vi "ArcadeDriveTest.vi"() -> ()   [LabVIEW 2013]
uses:
  <vilib>/Rock Robotics/WPI/Joystick/WPI_JoystickDeviceEnum.ctl
  <vilib>/Rock Robotics/SystemInterfaces/DIO/FPGA_DIOPWMChannel.ctl
  <vilib>/Rock Robotics/WPI/RobotDrive/WPI_RobotDriveOpen4MotorWithTalon.vi
  ArcadeDrivePieceWise.vi
  <vilib>/Rock Robotics/WPI/RobotDrive/WPI_RobotDriveArcadeDrive_RatioCurve.vi
panel:
  in  "Cutoff":dbl=0.7 format="%#_13g"
  in  "Deadzone":dbl=0.05 format="%#_13g"
  in  "UseWPILib?":bool
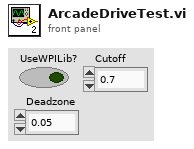
[diagram p1: front panel]
types:
  T1 = typedef "FPGA_DIOPWMChannel.ctl" = enum8{"PWM 1", "PWM 2", "PWM 3", "PWM 4", "PWM 5", "PWM 6", "PWM 7", "PWM 8", "PWM 9", "PWM 10", "Invalid"}
  T2 = typedef "WPI_JoystickDeviceEnum.ctl" = enum16{"USB 1", "USB 2", "USB 3", "USB 4", "Kinect 1", "Kinect 2"}
  T3 = typedef "WPI_RobotDriveDevRef.ctl" = cluster{"DevStatus":errorcluster, "Motors[]":T4[], "Square Inputs":bool, "Max Output":dbl, "Isochronous":bool}
  T4 = typedef "WPI_MotorControlDeviceRef.ctl" = cluster{"DeviceStatus":errorcluster, "Type":enum16{"PWM", "CAN"}, "PWM":cluster{"Digital Module":T5, "PWM Channel":T1, "DeadBand":T6}, "CAN":cluster{"Device Number":u8, "Control Mode":T7, "Semaphore":T8, "Max Vout":dbl}, "Invert":bool, "TransformRef":T9, "InvTransformRef":T9}
  T5 = typedef "FPGA_TypedefDigitalModule.ctl" = enum16{"Digital Module 1", "Digital Module 2"}
  T6 = typedef "WPI_PWMDeadband.ctl" = cluster{"Name":string, "maxPositivePwm":i32, "minPositivePwm":i32, "centerPwm":i32, "maxNegativePwm":i32, "minNegativePwm":i32, "angularRange":u16}
  T7 = typedef "WPI_CANJaguar_ControlMode.ctl" = enum8{"Percent VBus", "Current", "Speed", "Position", "Voltage"}
  T8 = typedef "Semaphore RefNum" = refnum<k1>
  T9 = typedef "WPI_PWMTransform_ConPane.ctl" = refnum<vi>
  T10 = typedef "WPI_JoystickDevRef.ctl" = cluster{"Device":T2}
  T11 = cluster{"axis 1 (x)":dbl, "axis 2 (y)":dbl, "axis 3 (throttle)":dbl, "axis 4":dbl, "axis 5":dbl, "axis 6":dbl}
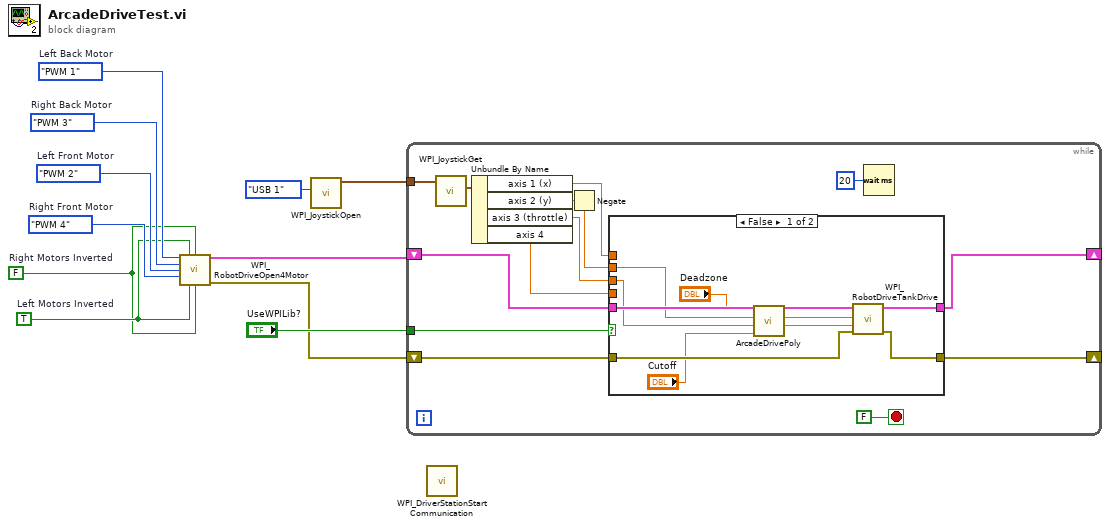
[diagram p0: block diagram]
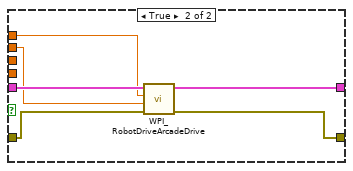
[diagram p2: hidden frame]
diagram:
  w5 = FPGA_DIOPWMChannel."PWM 4"  # Right Front Motor
  w6 = FPGA_DIOPWMChannel."PWM 2"  # Left Front Motor
  w7 = FPGA_DIOPWMChannel."PWM 3"  # Right Back Motor
  w8 = FPGA_DIOPWMChannel."PWM 1"  # Left Back Motor
  w3 = FALSE  # Right Motors Inverted
  w4 = TRUE  # Left Motors Inverted
  n1 = call-poly <vilib>:"WPI_RobotDriveOpen4Motor.vi"("Rear Left Motor"=w8, "Rear Left Motor Inverted"=w4, "Rear Right Motor Inverted"=w3, "Rear Right Motor"=w7, "Front Left Motor"=w6, "Front Right Motor"=w5, "Front Left Motor Inverted"=w4, "Front Right Motor Inverted"=w3) -> ("RobotDriveDevRef"=w2:T3, "error out"=w1:errorcluster)  [unwired: 6 in]
  n2 = call <vilib>:"WPI_JoystickOpen.vi"("JoystickDevice"=WPI_JoystickDeviceEnum."USB 1") -> ("JoystickDevRef"=w9:T10)  [unwired: 10 in]
  n3 = while {
    tunnel: "UseWPILib?" -> [w23]
    tunnel: w9 -> [w22]
    shift-right: [w14] -> _
    shift-left: w2 -> [w17]
    shift-right: [w15] -> _
    shift-left: w1 -> [w16]
    stop <- FALSE stop-if-true
    n4 = call <vilib>:"WPI_JoystickGet.vi"("JoystickDevRef"=w22) -> ("Axes"=w21:T11)  [unwired: 4 in, 2 out]
    n5 = Unbundle By Name(w21) -> ("axis 1 (x)"=w18:dbl, "axis 2 (y)"=w19:dbl, "axis 3 (throttle)"=w20:dbl, "axis 4"=w13:dbl)
    n6 = Negate(x=w19) -> (-x=w12:dbl)
    n7 = case shown="False" w23 {
      tunnel: w20 -> [w27 _]
      tunnel: w12 -> [w28 w40]
      tunnel: w18 -> [_ w39]
      tunnel: w17 -> [w35 w41]
      tunnel: w16 -> [w33 w38]
      tunnel: [w32 w37] -> w15
      tunnel: [w34 w36] -> w14
      tunnel: w13 -> [_ _]
      frame False {
        n8 = call-poly "ArcadeDrivePoly.vi"("Cutoff"="Cutoff", "Direction"=w27, "Throttle"=w28, "Deadzone"="Deadzone") -> ("DriveRight"=w29:dbl, "DriveLeft"=w30:dbl)  [unwired: 6 in]
        n9 = call <vilib>:"WPI_RobotDriveTankDrive.vi"("error in (no error)"=w33, "Right axis value"=w29, "Left axis value"=w30, "RobotDriveDevRef"=w35) -> ("error out"=w32:errorcluster, "RobotDriveDevRef"=w34:T3)  [unwired: 5 in, 1 out]
      }
      frame True {
        n10 = call-poly <vilib>:"WPI_RobotDriveArcadeDrive.vi"("error in (no error)"=w38, "Y axis value (Speed)"=w40, "X axis value (Curve)"=w39, "RobotDriveDevRef"=w41) -> ("error out"=w37:errorcluster, "RobotDriveDevRef"=w36:T3)  [unwired: 5 in, 1 out]
      }
    }
    n11 = Wait (ms)(milliseconds to wait=u32 20) -> ()  [unwired: 1 out]
  }
  n12 = call <vilib>:"WPI_DriverStationStart Communication.vi"() -> ()  [unwired: 12 in]
